vi "Rotate a point.vi"(7 "Gyro":dbl, 8 "Y":dbl, 11 "X":dbl) -> (0 "Y'":dbl, 3 "X'":dbl)   [LabVIEW 2018]
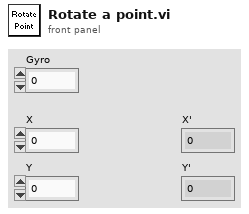
[diagram p1: front panel]
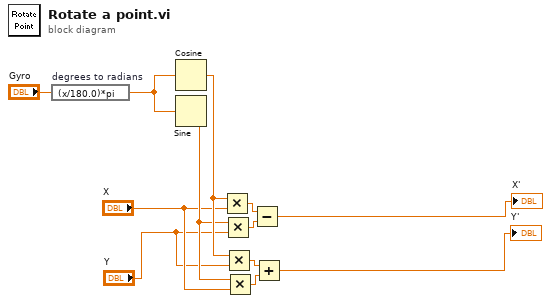
[diagram p0: block diagram]
diagram:
  n1 = expression code="(x/180.0)*pi" "degrees to radians"("Gyro") -> (w11:dbl)
  n2 = Cosine(x=w11) -> (cos(x)=w7:dbl)
  n3 = Sine(x=w11) -> (sin(x)=w6:dbl)
  n4 = Multiply(x=w7, y="X") -> (x*y=w10:dbl)
  n5 = Multiply(x=w6, y="Y") -> (x*y=w9:dbl)
  n6 = Multiply(x=w7, y="Y") -> (x*y=w3:dbl)
  n7 = Multiply(x=w6, y="X") -> (x*y=w2:dbl)
  n8 = Subtract(x=w10, y=w9) -> (x-y=→"X'":dbl)
  n9 = Add(x=w3, y=w2) -> (x+y=→"Y'":dbl)
